vi "Register Control Endpoint.vi"(6 "Endpoint Prefix (\"/c\")":string="/c", 7 "Endpoint Name (\"\"=Use Control Label)":string, 8 "Error In":errorcluster, 10 "Endpoint Access Mode (Read/Write)":T1=enum."Read/Write", 11 "Control Ref":refnum<vi>) -> (0 "Error Out":errorcluster)   [LabVIEW 2023, in "Server.lvclass"]
uses:
  Server.lvclass
  Control Ref Endpoint Access Mode.ctl
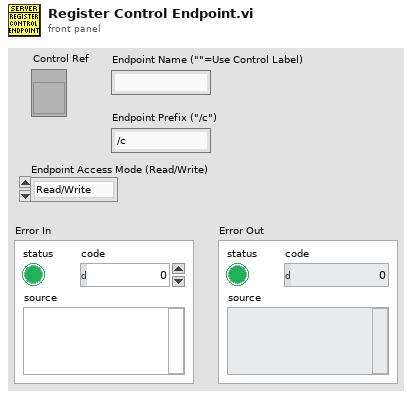
[diagram p1: front panel]
types:
  T1 = typedef "Server.lvclass/Control Ref Endpoint Access Mode.ctl" = enum16{"None", "Read/Write", "Read Only", "Write Only"}
  T2 = typedef "Server.lvclass/ObjectAttributes.ctl" = cluster{"Static Data":path, "MIME Types":variant, "Shutdown":bool, "API Queue":refnum<queue>, "ControlEndpoints":map{string, cluster{"Ref":refnum<vi>, "Mode":T3}}, "EventEndpoints":map{string, refnum<user-event>}}
  T3 = typedef "Control Ref Endpoint Access Mode.ctl" = enum16{"None", "Read/Write", "Read Only", "Write Only"}
  T4 = map{string, cluster{"Ref":refnum<vi>, "Mode":T3}}
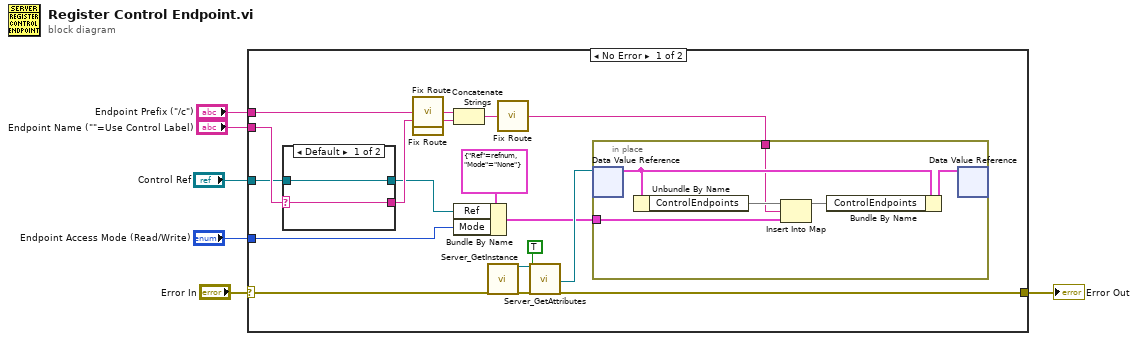
[diagram p0: block diagram]
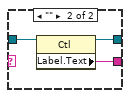
[diagram p2: hidden frame]
diagram:
  n1 = case shown="No Error" "Error In" {
    selector: "Error In" -> [w22 w36]
    tunnel: [w24 w36] -> w5
    tunnel: "Endpoint Prefix (\"/c\")" -> [w18 _]
    tunnel: "Endpoint Name (\"\"=Use Control Label)" -> [w16 _]
    tunnel: "Control Ref" -> [w15 _]
    tunnel: "Endpoint Access Mode (Read/Write)" -> [w9 _]
    frame No Error {
      n2 = case shown="Default" w16 {
        selector: w16 -> [w26 _]
        tunnel: w15 -> [w25 w29]
        tunnel: [w26 w28] -> w13
        tunnel: [w25 w27] -> w10
        frame Default {
        }
        frame "" {
          n3 = property class="Ctl"(reference=w29) -> (reference out=w27:refnum<vi>, "Label.Text"=w28:string)  [unwired: 1 in, 1 out]
        }
      }
      n4 = call "Fix Route.vi"("Route"=w18) -> ("Proper Route"=w17:string)
      n5 = call "Fix Route.vi"("Route"=w13) -> ("Proper Route"=w14:string)
      n6 = Concatenate Strings(w17, w14) -> (w8:string)
      n7 = Bundle By Name(cluster=cluster{"Ref":refnum<vi>, "Mode":T1} {"Ref"=refnum, "Mode"=enum."None"} ("value"), "Ref"=w10, "Mode"=w9) -> (w11:cluster{"Ref":refnum<vi>, "Mode":T1})
      n8 = call "Server_GetInstance.vi"("error in (no error)"=w22) -> ("reference out"=w23:refnum<class "Server.lvclass">, "error out"=w21:errorcluster)  [unwired: 14 in, 3 out]
      n9 = call "Fix Route.vi"("Route"=w8) -> ("Proper Route"=w7:string)
      n10 = call "Server_GetAttributes.vi"("reference in"=w23, "OnlyGetDvrReference(False)"=TRUE, "error in (no error)"=w21) -> ("DataRef"=w19:refnum<data-value>, "error out"=w24:errorcluster)  [unwired: 13 in, 2 out]
      n11 = in-place {
        in-place-border: w7 -> [w31]
        in-place-border: w11 -> [w30]
        n12 = in-place-dvr #1(w19) -> (w33:T2)  [unwired: 1 out]
        n13 = Unbundle By Name(w33) -> ("ControlEndpoints"=w35:T4)
        n14 = Insert Into Map(map in=w35, key=w31, value=w30) -> (map out=w34:T4)  [unwired: 2 out]
        n15 = Bundle By Name(cluster=w33, "ControlEndpoints"=w34) -> (w32:T2)
        n16 = in-place-dvr #1(w32) -> ()  [unwired: 2 out]
      }
    }
    frame Error {
    }
  }
  "Error Out" <- w5
